vi "Check Amplitude Bin.vi"(1 "Threshold Amp":dbl, 2 "Succ Max Amp":dbl, 3 "Max Amp":dbl, 4 "Prev Max Amp":dbl) -> (0 "Check Amp Ok?":bool)   [LabVIEW 2014]
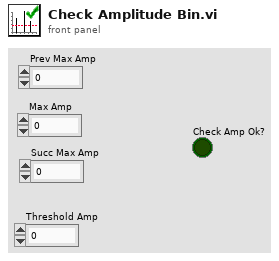
[diagram p1: front panel]
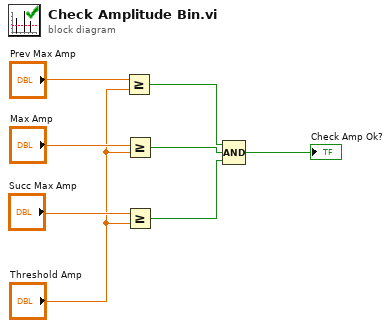
[diagram p0: block diagram]
diagram:
  n1 = Greater Or Equal?(x="Prev Max Amp", y="Threshold Amp") -> (x >= y?=w2:bool)
  n2 = Greater Or Equal?(x="Max Amp", y="Threshold Amp") -> (x >= y?=w3:bool)
  n3 = Greater Or Equal?(x="Succ Max Amp", y="Threshold Amp") -> (x >= y?=w4:bool)
  n4 = Compound Arithmetic op=AND(w2, w3, w4) -> (→"Check Amp Ok?":bool)
